vi "Stop Module.vi"(8 "error in (no error)":errorcluster, 11 "Wait for Stop Execution?":bool) -> (0 "error out":errorcluster, 3 "Response":string)   [LabVIEW 2015, in "Generic Module Library.lvlib" / "Template G_Module.lvlib"]
uses:
  Template G_Module.lvlib
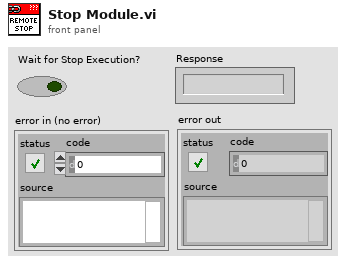
[diagram p1: front panel]
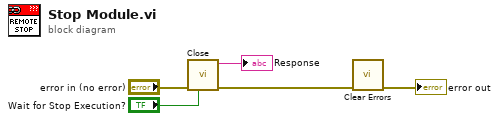
[diagram p0: block diagram]
diagram:
  n1 = call "Close.vi"("ACK"="Wait for Stop Execution?", "error in"="error in (no error)") -> ("error out"=w4:errorcluster, "Response"=→"Response":string)  [unwired: 8 in]
  n2 = call <vilib>:"Clear Errors.vi"("error in (no error)"=w4) -> ("error out"=→"error out":errorcluster)  [unwired: 5 in, 1 out]
